vi "Pressure Monitor Generate HK List.vi"() -> (2 "Channel Names":string[](array[string])=["Telescope RA", "Telescope DEC", "Telescope Moving?", "Telescope Status"], 3 "Channel List":refnum<class "HK Item.lvclass">[](array[class]))   [LabVIEW 2021]
uses:
  hk-channel-class/HK Item/HK Item.lvclass
  hk-channel-class/HK Item/HK Channel Units and Setup.ctl
  hk-channel-class/HK Item/HK Channel enum Data Type.ctl
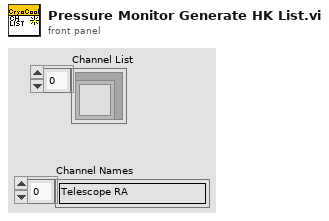
[diagram p1: front panel]
types:
  T1 = typedef "HK Item.lvclass/HK Channel Units and Setup.ctl" = cluster{"Unit Type":string, "Units":string, "Configuration":string, "Digits":i32, "Data Type":T2, "Exponential?":bool, "Source":string}
  T2 = typedef "HK Item.lvclass/HK Channel enum Data Type.ctl" = enum16{"Floating Point", "Integer", "Enum", "String", "Waveform", "File"}
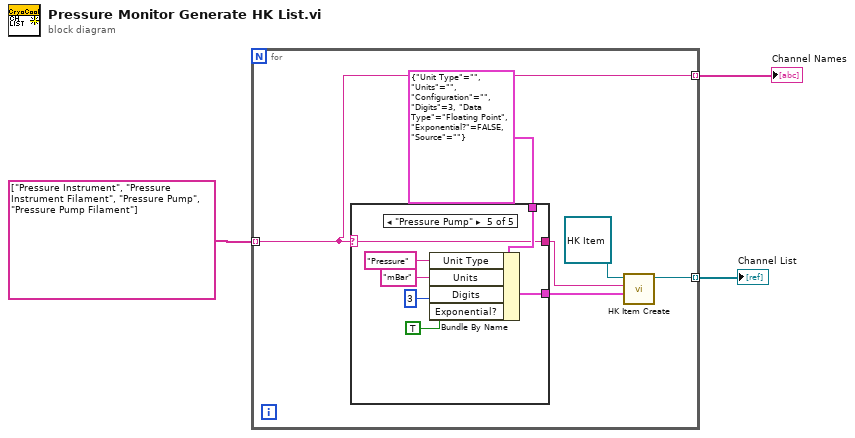
[diagram p0: block diagram]
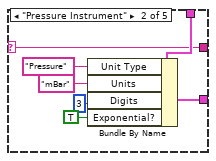
[diagram p3: hidden frame]
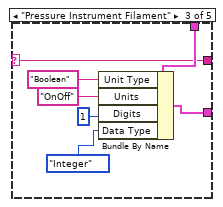
[diagram p4: hidden frame]
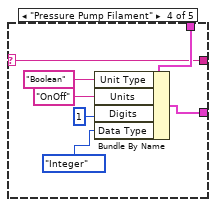
[diagram p5: hidden frame]
diagram:
  n1 = for {
    tunnel: string[] ["Pressure Instrument", "Pressure Instrument Filament", "Pressure Pump", "Pressure Pump Filament"] -> [w4] mode=indexing
    tunnel: [w6] -> w3 mode=indexing
    tunnel: [w4] -> w2 mode=indexing
    n2 = case shown="\"Pressure Pump\"" w4 {
      selector: w4 -> [w11 w13 w19 w26 w34]
      tunnel: T1 {"Unit Type"="", "Units"="", "Configuration"="", "Digits"=3, "Data Type"=enum."Floating Point", "Exponential?"=FALSE, "Source"=""} ("Channel Setup") -> [w10 w18 w25 w32 w39]
      tunnel: [w10 w14 w20 w27 w35] -> w9
      tunnel: [w11 w13 w19 w26 w34] -> w8
      frame "False", Default {
      }
      frame "Pressure Instrument" {
        n3 = Bundle By Name(cluster=w18, "Unit Type"="Pressure", "Units"="mBar", "Digits"=3, "Exponential?"=TRUE) -> (w14:T1)
      }
      frame "Pressure Instrument Filament" {
        n4 = Bundle By Name(cluster=w25, "Unit Type"="Boolean", "Units"="OnOff", "Digits"=1, "Data Type"=HK_Channel_enum_Data_Type."Integer") -> (w20:T1)
      }
      frame "Pressure Pump Filament" {
        n5 = Bundle By Name(cluster=w32, "Unit Type"="Boolean", "Units"="OnOff", "Digits"=1, "Data Type"=HK_Channel_enum_Data_Type."Integer") -> (w27:T1)
      }
      frame "Pressure Pump" {
        n6 = Bundle By Name(cluster=w39, "Unit Type"="Pressure", "Units"="mBar", "Digits"=3, "Exponential?"=TRUE) -> (w35:T1)
      }
    }
    n7 = call-dynamic "HK Item Create.vi"("Channel Setup"=w9, "Name"=w8, "HK Item in"=refnum<class "HK Item.lvclass"> refnum) -> ("HK Item out"=w6:refnum<class "HK Item.lvclass">)  [unwired: 7 in, 1 out]
  }
  "Channel List" <- w3
  "Channel Names" <- w2
